vi "Exp no 4a Half Adder.vi"() -> ()   [LabVIEW 2010]
panel:
  out "CARRY":bool
  out "SUM":bool
  in  "Y":bool
  in  "X":bool
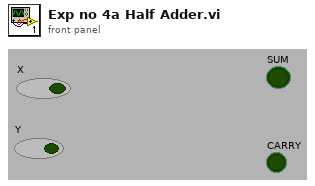
[diagram p1: front panel]
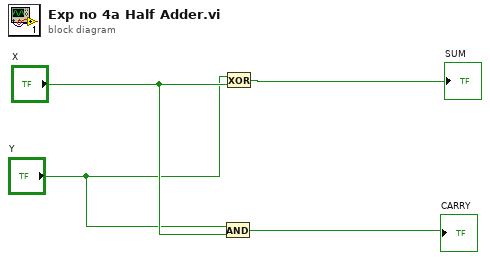
[diagram p0: block diagram]
diagram:
  n1 = And(x="Y", y="X") -> (x .and. y?=→"CARRY":bool)
  n2 = Exclusive Or(1:"X", 2:"Y") -> (0:→"SUM":bool)
